vi "xijk_select_best_filter_calculate_ratio.vi"(7 "spectra parameters in":T1={"Booleans"={"Unknown detector"=FALSE, "Dual band filters"=FALSE, "Dual emission by cubes"=FALSE, "FRET"=FALSE}, "Integers"={"Light source"=0, "Number of fluorophores"=0, "Wavelength of laser (nm) 1"=0, "Broadness of laser (nm) 1"=0.0, "Wavelength of laser (nm) 2"=0, "Broadness of laser (nm) 2"=0.0, "Template"=1}, "Doubles"={"Molar extinction 1"=1.0, "Molar extinction 2"=1.0, "Quantum efficiency 1"=1.0, "Quantum efficiency 2"=1.0}}, 10 "calculation table":i32[](array[numeric])=[8, 15, 13, 10], 11 "all rows":string[][](array[string]) caption="toutes les lignes") -> (3 "all rows out":string[][](array[string]))   [LabVIEW 2009, in "xijk_select_best_filter.lvlib"]
uses:
  xijk_select_best_filter.lvlib
  Type Def/spectra_parameters.ctl
panel:
  out "Array 4":dbl[](array[numeric])
  out "Array 3":dbl[](array[numeric])
  out "Array 2":dbl[](array[numeric])
  out "Array":dbl[](array[numeric])
  in  "y":dbl=1.5
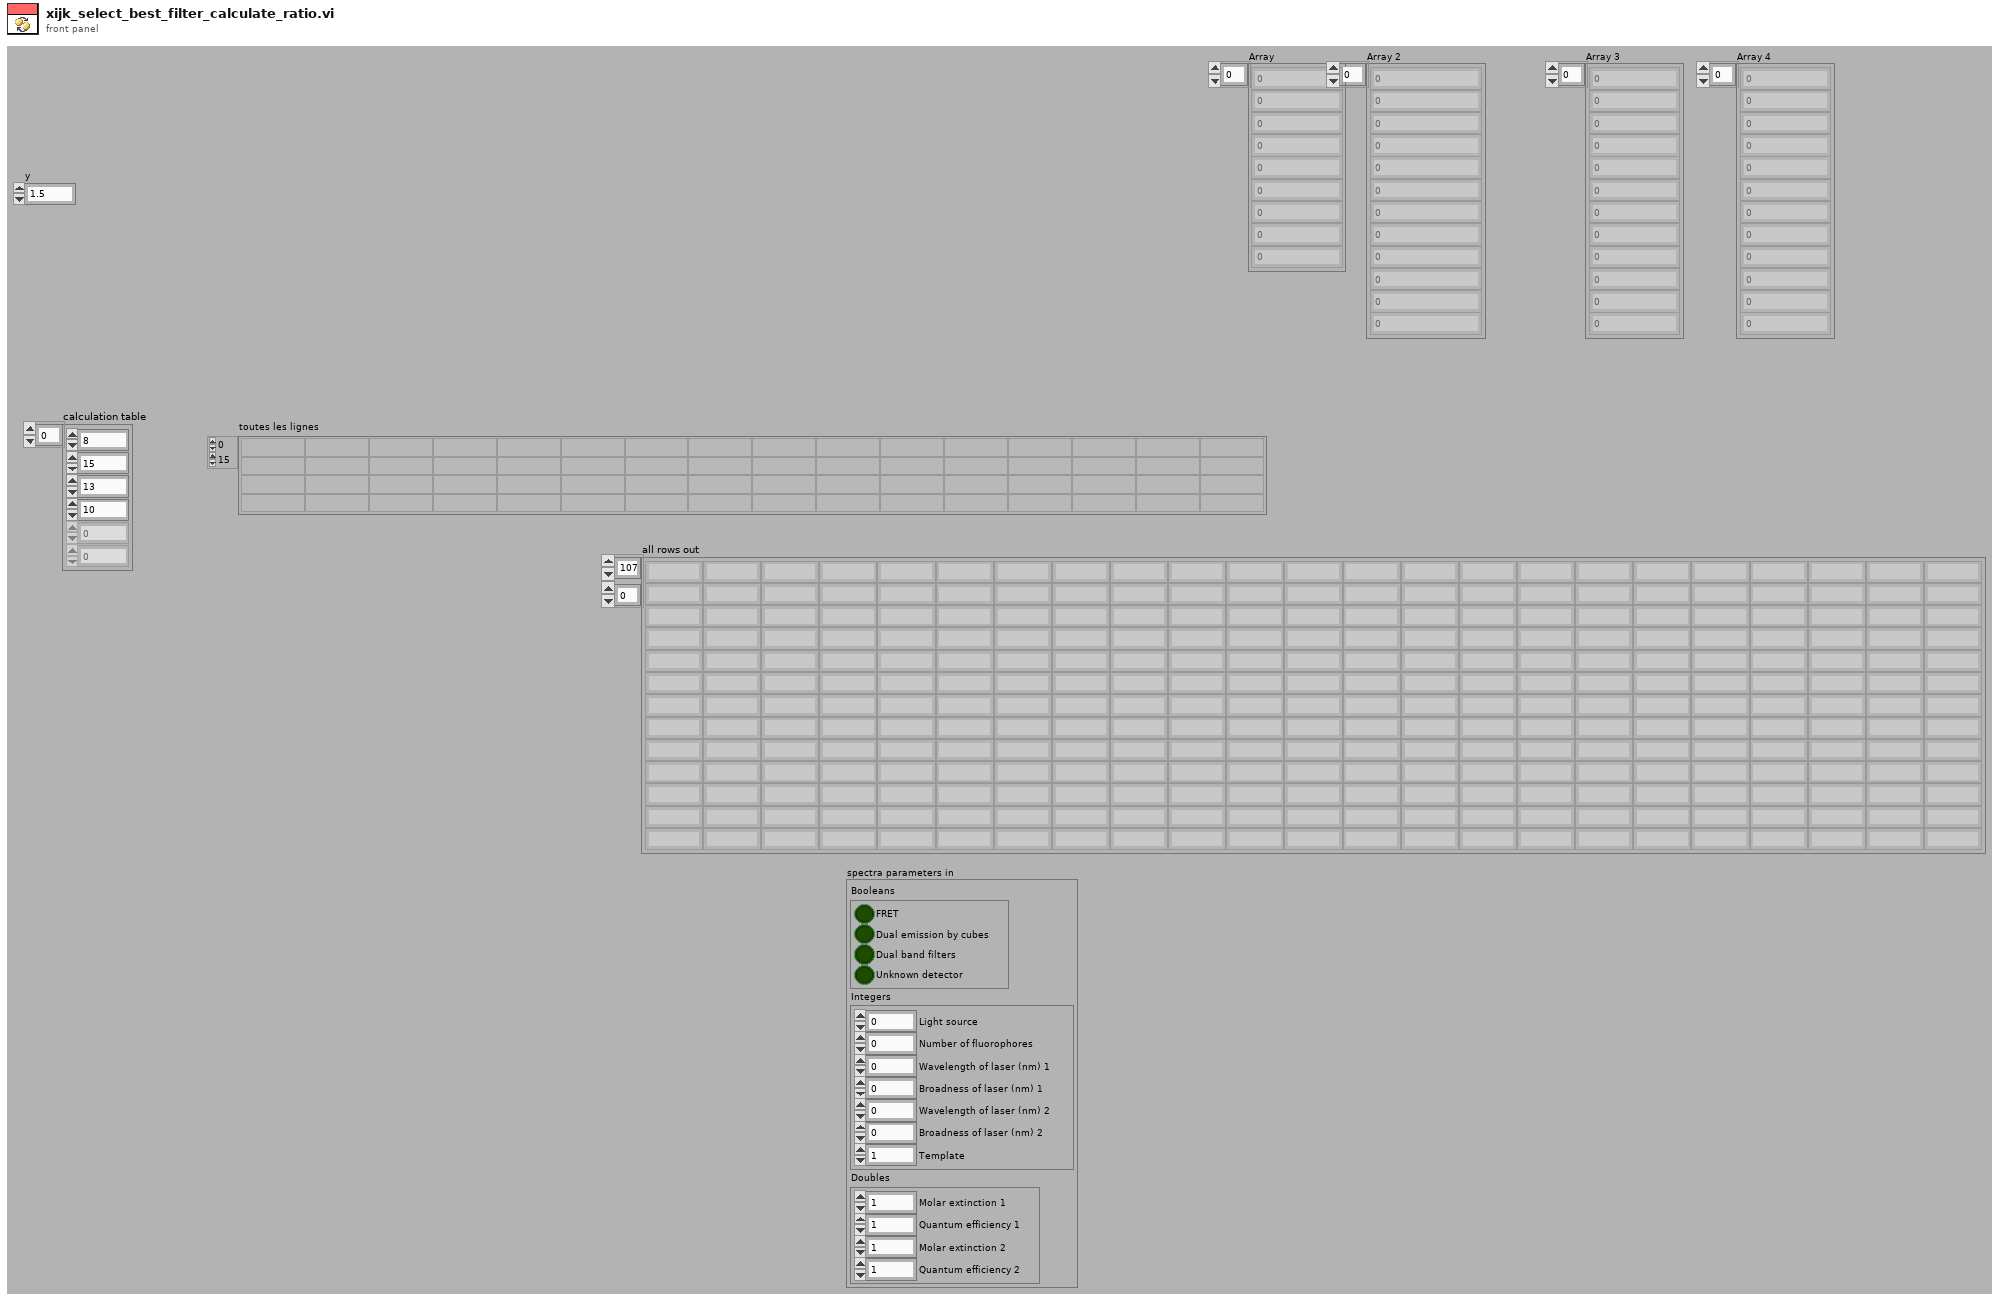
[diagram p1: front panel]
types:
  T1 = typedef "spectra_parameters.ctl" = cluster{"Booleans":cluster{"Unknown detector":bool, "Dual band filters":bool, "Dual emission by cubes":bool, "FRET":bool}, "Integers":cluster{"Light source":u16, "Number of fluorophores":u16, "Wavelength of laser (nm) 1":u16, "Broadness of laser (nm) 1":sgl, "Wavelength of laser (nm) 2":u16, "Broadness of laser (nm) 2":sgl, "Template":u16}, "Doubles":cluster{"Molar extinction 1":sgl, "Molar extinction 2":sgl, "Quantum efficiency 1":sgl, "Quantum efficiency 2":sgl}}
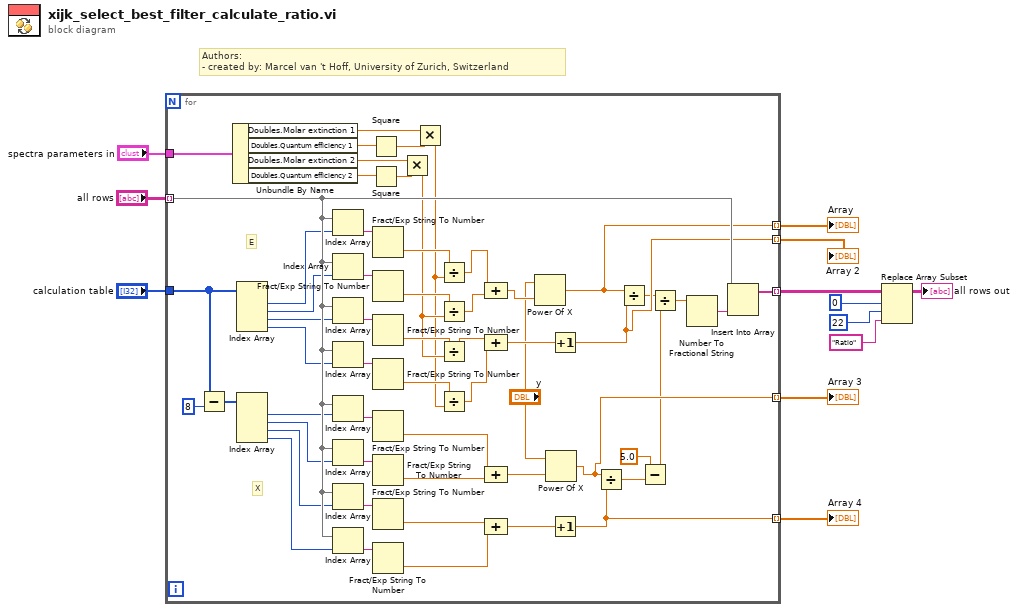
[diagram p0: block diagram]
diagram:
  # "Authors: \n- created by: Marcel van 't Hoff, University of Zurich, Switzerland"
  n1 = for {
    tunnel: "all rows" -> [w67] mode=indexing
    tunnel: [w68] -> w7 mode=indexing
    tunnel: "calculation table" -> [w66]
    tunnel: [w64] -> w5 mode=indexing
    tunnel: [w63] -> w4 mode=indexing
    tunnel: [w62] -> w3 mode=indexing
    tunnel: [w61] -> w2 mode=indexing
    tunnel: "spectra parameters in" -> [w29]
    # "X"
    # "E"
    n2 = Subtract(x=w66, y=8 ("indice")) -> (x-y=w41:i32[])
    n3 = Unbundle By Name(w29) -> ("Doubles.Molar extinction 1"=w27:sgl, "Doubles.Quantum efficiency 1"=w28:sgl, "Doubles.Molar extinction 2"=w24:sgl, "Doubles.Quantum efficiency 2"=w25:sgl)
    n4 = Index Array(array=w66) -> (element #1=w55:i32, element #2=w56:i32, element #3=w54:i32, element #4=w53:i32)  [unwired: 4 in]
    n5 = Index Array(array=w41) -> (element #1=w40:i32, element #2=w39:i32, element #3=w38:i32, element #4=w37:i32)  [unwired: 4 in]
    n6 = Index Array(array=w67, index=w55) -> (element=w59:string)
    n7 = Index Array(array=w67, index=w56) -> (element=w60:string)
    n8 = Index Array(array=w67, index=w54) -> (element=w58:string)
    n9 = Index Array(array=w67, index=w53) -> (element=w57:string)
    n10 = Index Array(array=w67, index=w40) -> (element=w47:string)
    n11 = Index Array(array=w67, index=w39) -> (element=w46:string)
    n12 = Index Array(array=w67, index=w38) -> (element=w45:string)
    n13 = Index Array(array=w67, index=w37) -> (element=w44:string)
    n14 = Square(x=w28) -> (x^2=w26:sgl)
    n15 = Square(x=w25) -> (x^2=w23:sgl)
    n16 = Fract/Exp String To Number(string=w59) -> (number=w20:dbl)  [unwired: 4 out]
    n17 = Fract/Exp String To Number(string=w60) -> (number=w22:dbl)  [unwired: 4 out]
    n18 = Fract/Exp String To Number(string=w58) -> (number=w18:dbl)  [unwired: 4 out]
    n19 = Fract/Exp String To Number(string=w57) -> (number=w16:dbl)  [unwired: 4 out]
    n20 = Fract/Exp String To Number(string=w47) -> (number=w50:dbl)  [unwired: 4 out]
    n21 = Fract/Exp String To Number(string=w46) -> (number=w51:dbl)  [unwired: 4 out]
    n22 = Fract/Exp String To Number(string=w45) -> (number=w49:dbl)  [unwired: 4 out]
    n23 = Fract/Exp String To Number(string=w44) -> (number=w48:dbl)  [unwired: 4 out]
    n24 = Multiply(x=w24, y=w23) -> (x*y=w14:sgl)
    n25 = Multiply(x=w27, y=w26) -> (x*y=w13:sgl)
    n26 = Divide(x=w20, y=w13) -> (x/y=w19:dbl)
    n27 = Divide(x=w22, y=w14) -> (x/y=w21:dbl)
    n28 = Divide(x=w18, y=w14) -> (x/y=w17:dbl)
    n29 = Divide(x=w16, y=w13) -> (x/y=w15:dbl)
    n30 = Compound Arithmetic op=ADD(w19, w21) -> (w33:dbl)
    n31 = Compound Arithmetic op=ADD(w17, w15) -> (w52:dbl)
    n32 = Compound Arithmetic op=ADD(w50, w51) -> (w32:dbl)
    n33 = Compound Arithmetic op=ADD(w49, w48) -> (w43:dbl)
    n34 = Power Of X(1:w33, 2:"y") -> (0:w64:dbl)
    n35 = Power Of X(1:w32, 2:"y") -> (0:w62:dbl)
    n36 = Increment(x=w52) -> (x+1=w63:dbl)
    n37 = Increment(x=w43) -> (x+1=w61:dbl)
    n38 = Divide(x=w62, y=w61) -> (x/y=w35:dbl)
    n39 = Divide(x=w64, y=w63) -> (x/y=w30:dbl)
    n40 = Subtract(x=5.0, y=w35) -> (x-y=w34:dbl)
    n41 = Divide(x=w30, y=w34) -> (x/y=w65:dbl)
    n42 = Number To Fractional String(number=w65) -> (F-format string=w69:string)  [unwired: 3 out]
    n43 = Insert Into Array(array=w67, new element=w69) -> (w68:string[])  [unwired: 1 in]
  }
  "Array" <- w5
  "Array 2" <- w4
  "Array 3" <- w3
  "Array 4" <- w2
  n44 = Replace Array Subset(array=w7, new element="Ratio" ("nouvel élément/sous-tableau"), index (row)=0 ("indice (ligne)"), index (col)=22 ("indice désactivé (col)")) -> (→"all rows out":string[][])
